vi "Check for Valid Host Interface.vi"(8 "error in (no error)":errorcluster, 11 "UniCyRO_Host_Sim in":refnum<class "UniCyRO_Host_Sim.lvclass">) -> (0 "error out":errorcluster, 2 "valid?":bool, 3 "UniCyRO_Host_Sim out":refnum<class "UniCyRO_Host_Sim.lvclass">)   [LabVIEW 2012, in "UniCyRO.lvlib" / "UniCyRO_Host_Sim.lvclass"]
uses:
  UniCyRO_Host_Sim.lvclass
  UniCyRO_Host_Sim.lvclass/UniCyRO_Host_Sim.ctl
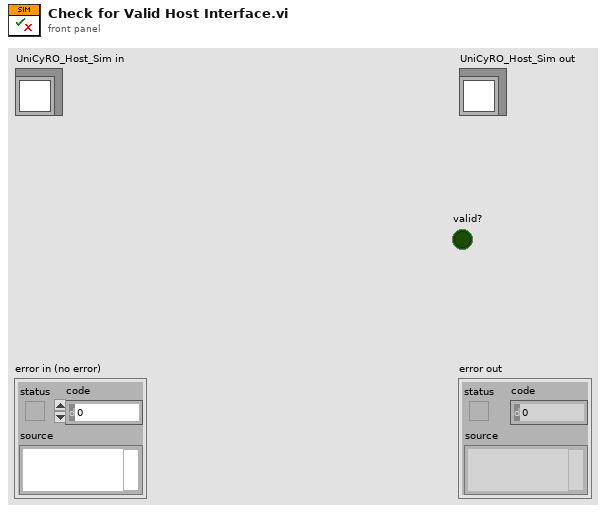
[diagram p1: front panel]
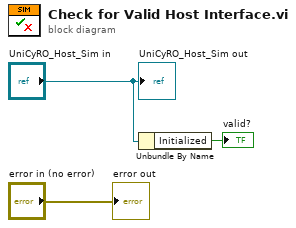
[diagram p0: block diagram]
diagram:
  n1 = Unbundle By Name("UniCyRO_Host_Sim in") -> ("Initialized"=→"valid?":bool)
  "error out" <- "error in (no error)"
  "UniCyRO_Host_Sim out" <- "UniCyRO_Host_Sim in"
